vi "main.vi"() -> ()   [LabVIEW 2012]
panel:
  out "Data over Time":cluster{"token":i32, "token":i32, "z":dbl}(graph)
  out "APRS Stream":string
  in  "Tab Control":enum32{"Tracking", "Settings"}(tab)
  out "Altitude in Feet":dbl(slide) scale=0.0..100000.0
  out "Humidity":dbl(knob) scale=0.0..100.0
  out "Outside Temp":i32(slide) scale=-100.0..100.0
  out "Inside Temp":i32(slide) scale=-100.0..100.0
  out "Login Status":bool=TRUE
  out "Link Status":bool=TRUE
  in  "stop":bool
  in  "server":string="rotate.aprs.net"
  in  "port":dbl=14580.0
  in  "Login":string="KE5GDB"
  in  "Password":string="18850"
  in  "Callsign for Tracking":string="K5UTD-4"
  out "Fleam Drive Monitor":bool[][](array[boolean])
  out "Poll Status":bool=TRUE
  # "Server Properties"
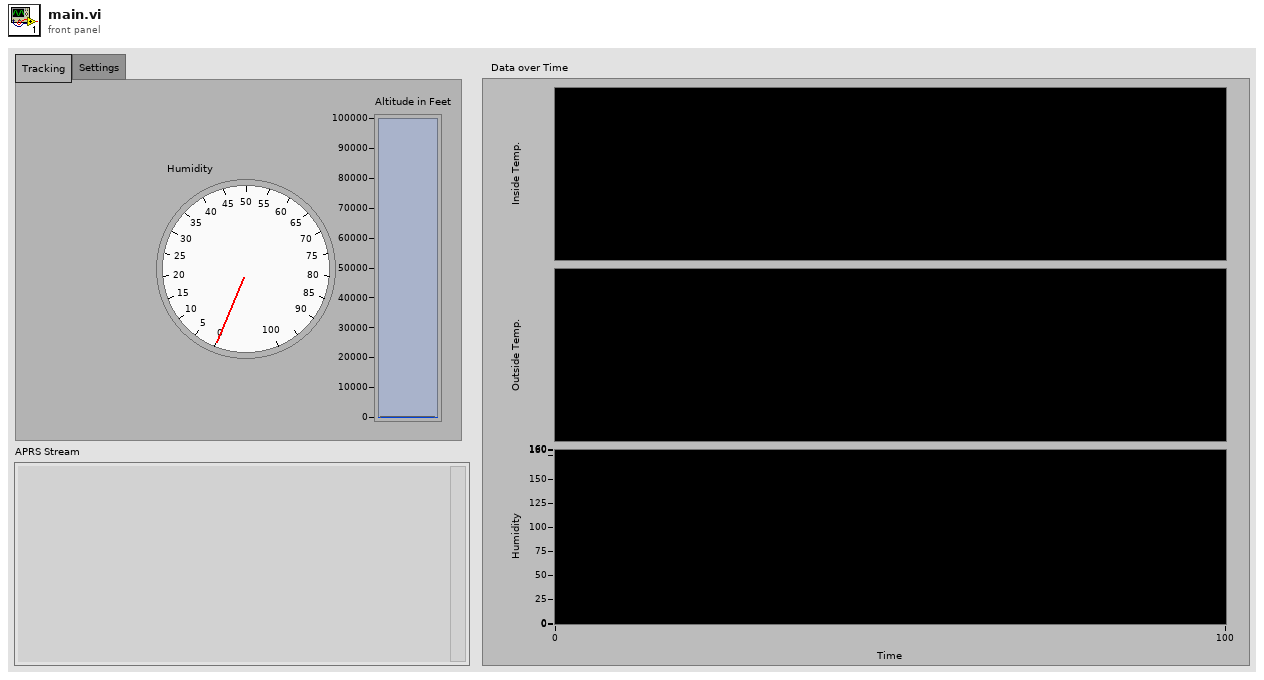
[diagram p1: front panel]
types:
  T1 = cluster{"connection ID":refnum<k5>, "login string":string, "callsign for filter":string}
  T2 = enum32{"invalid app kind", "Development System", "Run Time System", "Student Edition", "Embedded LabVIEW", "Evaluation", "Custom"}
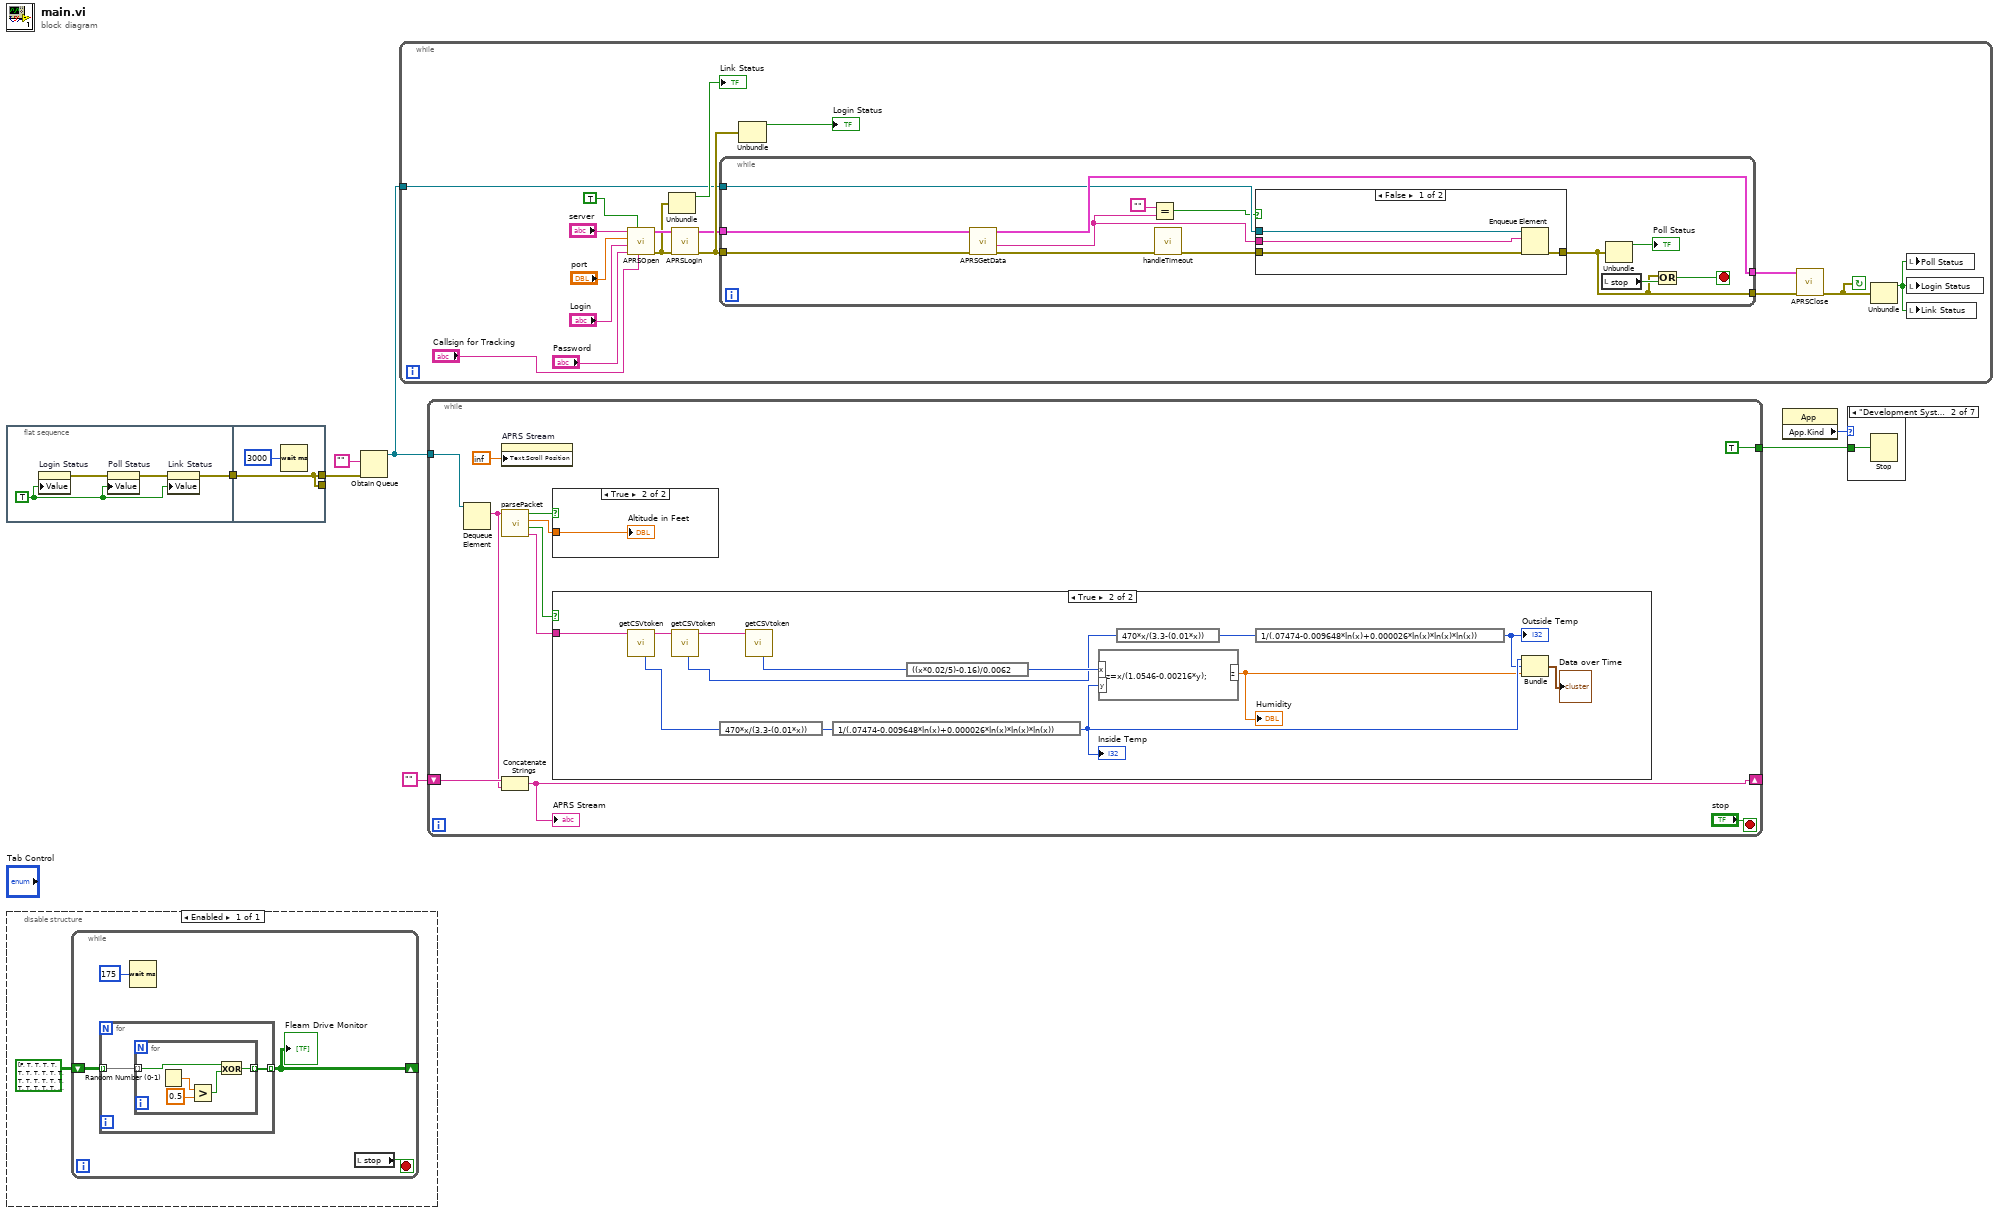
[diagram p0: block diagram]
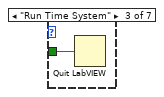
[diagram p3: hidden frame]
diagram:
  n1 = flat-sequence {
    tunnel: [w8] -> w7
    tunnel: [w12] -> _
    tunnel: w7 -> [w12]
    tunnel: [w12] -> w3
    frame #0 {
      w11 = TRUE
      n2 = property on="Login Status" class="Bool (strict)"("Value"=w11) -> (error out=w10:errorcluster)  [unwired: 2 in, 1 out]
      n3 = property on="Poll Status" class="Bool (strict)"(error in=w10, "Value"=w11) -> (error out=w9:errorcluster)  [unwired: 1 in, 1 out]
      n4 = property on="Link Status" class="Bool (strict)"(error in=w9, "Value"=w11) -> (error out=w8:errorcluster)  [unwired: 1 in, 1 out]
    }
    frame #1 {
      n5 = Wait (ms)(milliseconds to wait=u32 3000) -> ()  [unwired: 1 out]
    }
  }
  n6 = disable-structure shown="Enabled" {
    frame Enabled {
      n7 = while {
        shift-right: [w17] -> _
        shift-left: bool[][] [[FALSE, TRUE, TRUE, TRUE, TRUE, TRUE, TRUE, TRUE, TRUE, TRUE, TRUE, TRUE, TRUE, TRUE, TRUE, TRUE, TRUE, TRUE, TRUE, TRUE], [TRUE, TRUE, TRUE, TRUE, TRUE, TRUE, TRUE, TRUE, TRUE, TRUE, TRUE, TRUE, TRUE, TRUE, TRUE, TRUE, TRUE, TRUE, TRUE, TRUE], [TRUE, TRUE, TRUE, TRUE, TRUE, TRUE, TRUE, TRUE, TRUE, TRUE, TRUE, TRUE, TRUE, TRUE, TRUE, TRUE, TRUE, TRUE, TRUE, TRUE], [TRUE, TRUE, TRUE, TRUE, TRUE, TRUE, TRUE, TRUE, TRUE, TRUE, TRUE, TRUE, TRUE, TRUE, TRUE, TRUE, TRUE, TRUE, TRUE, TRUE], [TRUE, TRUE, TRUE, TRUE, TRUE, TRUE, TRUE, TRUE, TRUE, TRUE, TRUE, TRUE, TRUE, TRUE, TRUE, TRUE, TRUE, TRUE, TRUE, TRUE], [TRUE, TRUE, TRUE, TRUE, TRUE, TRUE, TRUE, TRUE, TRUE, TRUE, TRUE, TRUE, TRUE, TRUE, TRUE, TRUE, TRUE, TRUE, TRUE, TRUE], [TRUE, TRUE, TRUE, TRUE, TRUE, TRUE, TRUE, TRUE, TRUE, TRUE, TRUE, TRUE, TRUE, TRUE, TRUE, TRUE, TRUE, TRUE, TRUE, TRUE], [TRUE, TRUE, TRUE, TRUE, TRUE, TRUE, TRUE, TRUE, TRUE, TRUE, TRUE, TRUE, TRUE, TRUE, TRUE, TRUE, TRUE, TRUE, TRUE, TRUE], [TRUE, TRUE, TRUE, TRUE, TRUE, TRUE, TRUE, TRUE, TRUE, TRUE, TRUE, TRUE, TRUE, TRUE, TRUE, TRUE, TRUE, TRUE, TRUE, TRUE], [TRUE, TRUE, TRUE, TRUE, TRUE, TRUE, TRUE, TRUE, TRUE, TRUE, TRUE, TRUE, TRUE, TRUE, TRUE, TRUE, TRUE, TRUE, TRUE, FALSE]] -> [w18]
        stop <- w15 stop-if-true
        n8 = for {
          tunnel: w18 -> [w20] mode=indexing
          tunnel: [w19] -> w17 mode=indexing
          n9 = for {
            tunnel: w20 -> [w22] mode=indexing
            tunnel: [w21] -> w19 mode=indexing
            n10 = Random Number (0-1)() -> (number: 0 to 1=w24:dbl)
            n11 = Greater?(x=w24, y=0.5) -> (0:w23:bool)
            n12 = Exclusive Or(1:w23, 2:w22) -> (0:w21:bool)
          }
        }
        "Fleam Drive Monitor" <- w17
        n13 = Wait (ms)(milliseconds to wait=u32 175) -> ()  [unwired: 1 out]
        n14 = local read "stop"() -> (w15:bool)
      }
    }
  }
  n15 = Obtain Queue(element data type="", error in (no error)=w3) -> (queue out=w4:refnum<queue>)  [unwired: 3 in, 2 out]
  n16 = while {
    tunnel: w4 -> [w26]
    stop <- w27 continue-if-true
    n17 = call "APRSOpen.vi"("callsign for filter"="Callsign for Tracking", "filter?"=TRUE ("attempt to filter"), "Password"="Password", "Login"="Login", "port"="port", "server"="server") -> ("error IO"=w35:errorcluster, "conRef"=w36:T1)  [unwired: 4 in]
    n18 = Unbundle(w35) -> ("status"=→"Link Status":bool)  [unwired: 2 out]
    n19 = call "APRSLogin.vi"("error in (no error)"=w35, "conRef"=w36) -> ("error out"=w34:errorcluster, "conRef out"=w29:T1)  [unwired: 8 in]
    n20 = while {
      tunnel: w34 -> [w53]
      tunnel: [w46] -> w31
      tunnel: [w52] -> w30
      tunnel: w29 -> [w51]
      tunnel: w26 -> [w48]
      stop <- w49 stop-if-true
      n21 = call "APRSGetData.vi"("error in (no error)"=w53, "conRef"=w51) -> ("error out"=w54:errorcluster, "APRS packet"=w43:string, "conRef out"=w52:T1)  [unwired: 7 in]
      n22 = Equal?(x="", y=w43) -> (x = y?=w44:bool)
      n23 = call "handleTimeout.vi"("error in (no error)"=w54) -> ("error out"=w47:errorcluster)  [unwired: 10 in]
      n24 = case shown="False" w44 {
        tunnel: w48 -> [w59 _]
        tunnel: w47 -> [w58 w60]
        tunnel: [w57 w60] -> w46
        tunnel: w43 -> [w56 _]
        frame False {
          n25 = Enqueue Element(queue=w59, element=w56, error in (no error)=w58) -> (error out=w57:errorcluster)  [unwired: 1 in, 2 out]
        }
        frame True {
        }
      }
      n26 = local read "stop"() -> (w50:bool)
      n27 = Unbundle(w46) -> ("status"=→"Poll Status":bool)  [unwired: 2 out]
      n28 = Or(x=w46, y=w50) -> (x .or. y?=w49:bool)
    }
    n29 = Unbundle(w34) -> ("status"=→"Login Status":bool)  [unwired: 2 out]
    n30 = call "APRSClose.vi"("error in (no error)"=w31, "conRef"=w30) -> ("error out"=w27:errorcluster)  [unwired: 9 in]
    n31 = Unbundle(w27) -> ("status"=w28:bool)  [unwired: 2 out]
    n32 = local write "Poll Status"(w28) -> ()
    n33 = local write "Login Status"(w28) -> ()
    n34 = local write "Link Status"(w28) -> ()
  }
  n35 = while {
    shift-right: [w71] -> _
    shift-left: "" -> [w70]
    tunnel: w4 -> [w68]
    tunnel: [TRUE] -> w1
    stop <- "stop" stop-if-true
    n36 = Dequeue Element(queue=w68) -> (element=w67:string)  [unwired: 2 in, 3 out]
    n37 = property on="APRS Stream" class="Str"("Text.Scroll Position"=inf) -> ()  [unwired: 2 in, 2 out]
    n38 = call "parsePacket.vi"("APRS Packet"=w67) -> (0:"Token String"=w66:string, 1:"Token String"=w63:bool, 2:"Altitude"=w64:dbl, 3:"Altitude"=w62:bool)  [unwired: 3 in]
    n39 = Concatenate Strings(w70, w67) -> (w71:string)
    "APRS Stream" <- w71
    n40 = case shown="True" w62 {
      tunnel: w64 -> [_ w72]
      frame False {
      }
      frame True {
        "Altitude in Feet" <- w72
      }
    }
    n41 = case shown="True" w63 {
      tunnel: w66 -> [_ w82]
      frame False {
      }
      frame True {
        n42 = call "getCSVtoken.vi"("packet string"=w82) -> ("remainder of packet"=w85:string, "token"=w78:i32)  [unwired: 9 in]
        n43 = call "getCSVtoken.vi"("packet string"=w85) -> ("remainder of packet"=w84:string, "token"=w77:i32)  [unwired: 9 in]
        n44 = expression code="470*x/(3.3-(0.01*x))"(w78) -> (w80:i32)
        n45 = call "getCSVtoken.vi"("packet string"=w84) -> ("token"=w76:i32)  [unwired: 9 in, 1 out]
        n46 = expression code="1/(.07474-0.009648*ln(x)+0.000026*ln(x)*ln(x)*ln(x))"(w80) -> (w75:i32)
        "Inside Temp" <- w75
        n47 = expression code="((x*0.02/5)-0.16)/0.0062"(w76) -> (w79:i32)
        n48 = formula code="z=x/(1.0546-0.00216*y);"("x"=w79, "y"=w75) -> ("z"=w73:dbl)
        "Humidity" <- w73
        n49 = expression code="470*x/(3.3-(0.01*x))"(w77) -> (w81:i32)
        n50 = expression code="1/(.07474-0.009648*ln(x)+0.000026*ln(x)*ln(x)*ln(x))"(w81) -> (w74:i32)
        "Outside Temp" <- w74
        n51 = Bundle("token"=w75, "token"=w74, "z"=w73) -> (→"Data over Time":cluster{"token":i32, "token":i32, "z":dbl})  [unwired: 1 in]
      }
    }
  }
  n52 = property class="App"() -> ("App.Kind"=w2:T2)  [unwired: 2 in, 2 out]
  n53 = case shown="\"Development System\"" w2 {
    tunnel: w1 -> [_ w86 w87 _ _ _ _]
    frame "invalid app kind", Default {
    }
    frame "Development System" {
      n54 = Stop(stop? (T)=w86) -> ()
    }
    frame "Run Time System" {
      n55 = Quit LabVIEW(quit? (T)=w87) -> ()
    }
    frame "Student Edition" {
    }
    frame "Embedded LabVIEW" {
    }
    frame "Evaluation" {
    }
    frame "Custom" {
    }
  }
